vi "Get Server.vi"(8 "error in (no error)":errorcluster, 11 "Method":enum16{"Get Server", "Close Server"}(ring)) -> (0 "error out":errorcluster, 3 "Server out":refnum<class "Server.lvclass">)   [LabVIEW 2024, in "Ramses Framework.lvlib" / "Server.lvclass"]
uses:
  Server.lvclass
  Server.lvclass/Server.ctl
  Read Server Running.vi
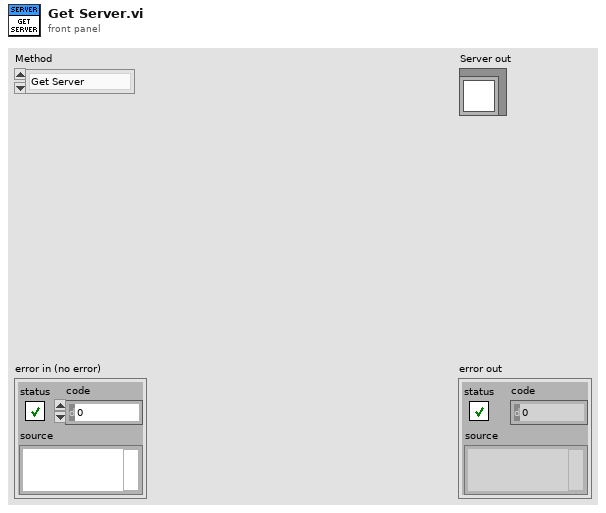
[diagram p1: front panel]
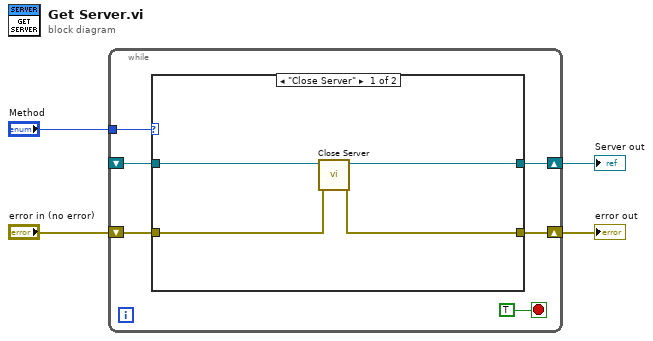
[diagram p0: block diagram]
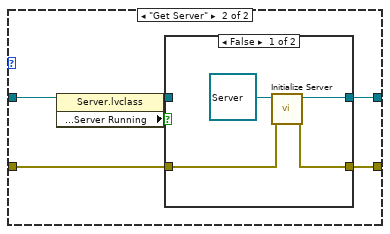
[diagram p2: hidden frame]
diagram:
  n1 = while {
    shift-right: [w7] -> w2
    shift-left: _ -> [w9]
    shift-right: [w6] -> w4
    shift-left: "error in (no error)" -> [w8]
    tunnel: "Method" -> [w5]
    stop <- TRUE stop-if-true
    n2 = case shown="\"Close Server\"" w5 {
      tunnel: w9 -> [w14 w20]
      tunnel: w8 -> [w13 w18]
      tunnel: [w11 w16] -> w7
      tunnel: [w12 w15] -> w6
      frame "Close Server" {
        n3 = call "Close Server.vi"("error in (no error)"=w13, "Base Server in"=w14) -> ("error out"=w12:errorcluster, "Base Server out"=w11:refnum<class "Server.lvclass">)  [unwired: 8 in]
      }
      frame "Get Server" {
        n4 = property class="Server.lvclass"(reference=w20) -> (reference out=w17:refnum<class "Server.lvclass">, "Public API:Accessors:Server Running"=w19:bool)  [unwired: 1 in, 1 out]
        n5 = case shown="False" w19 {
          tunnel: w18 -> [w23 w25]
          tunnel: w17 -> [_ w26]
          tunnel: [w24 w26] -> w16
          tunnel: [w22 w25] -> w15
          frame False {
            n6 = call "Initialize Server.vi"("error in (no error)"=w23, "Base Server in"=refnum<class "Server.lvclass"> refnum) -> ("error out"=w22:errorcluster, "Base Server out"=w24:refnum<class "Server.lvclass">)  [unwired: 8 in]
          }
          frame True {
          }
        }
      }
    }
  }
  "error out" <- w4
  "Server out" <- w2
